vi "KI6221.vi"() -> ()   [LabVIEW 2019] (continued)
      w132 = u16 5 ("Measure Connect LAST")
      w116 = FALSE ("Visible")
      w129 = 0 ("Numeric 2")
      # "SHOW HELP"
      # "Makes 6220 pic NOT visible,\nbecause we don't yet have a\npic... Change with graphics."
      # "Clear setup WIzard"
      n79 = local read "Select the current source model number:"() -> (w119:u16)
      n80 = property on="Verify instruments" class="Bool (strict)"("Visible"=w116) -> ()  [unwired: 2 in, 2 out]
      n81 = property on="BIG DISP OVERLAY" class="Bool (strict)"("Caption.Visible"=w116) -> ()  [unwired: 2 in, 2 out]
      n82 = property on="DUT connect HELP" class="Bool"("Visible"=w116) -> ()  [unwired: 2 in, 2 out]
      n83 = Not(x=w116) -> (.not. x?=w138:bool)
      n84 = property on="DC TABS" class="TabCtl (strict)" props=["Pages", "Value"]() -> (error out=w134:errorcluster, "Pages"=w137:refnum<vi>[])  [unwired: 2 in, 2 out]
      n85 = local read "Power:"() -> (w121:u16)
      n86 = case shown="1" w121 {
        frame 0, Default {
          n87 = local write "INCREMENT"(16.666667) -> ()
        }
        frame 1 {
          n88 = local write "INCREMENT"(20.0) -> ()
        }
      }
      n89 = property on="Voltage\n Compliance" class="DigNum (strict)"("Disabled"=w122) -> ()  [unwired: 2 in, 2 out]
      n90 = property on="SAVE 2" class="Bool"("Disabled"=w129) -> ()  [unwired: 2 in, 2 out]
      n91 = property on="Signal Repetition \nFrequency (Hz)" class="DigNum (strict)"("Disabled"=w122) -> ()  [unwired: 2 in, 2 out]
      n92 = property on="NEW INSTR SETUP" class="Bool"("Disabled"=w129) -> ()  [unwired: 2 in, 2 out]
      n93 = property on="WEB UPDATES" class="Bool (strict)"("Disabled"=w129) -> ()  [unwired: 2 in, 2 out]
      n94 = property on="OPEN" class="Bool (strict)"("Disabled"=w129) -> ()  [unwired: 2 in, 2 out]
      n95 = property on="GENERATE SCPI - ADVANCED" class="Bool"("Disabled"=w129) -> ()  [unwired: 2 in, 2 out]
      n96 = invoke on="Main intro bar" class="Picture" method="Reinit To Default"() -> ()  [unwired: 3 in, 3 out]
      n97 = property on="waveform tabs 2" class="TabCtl (strict)"("Disabled"=w122) -> ()  [unwired: 2 in, 2 out]
      n98 = property on="Waveform Type" class="Ring (strict)"("Disabled"=w122) -> ()  [unwired: 2 in, 2 out]
      n99 = property on="______________________________________________________________________________________________________________" class="Bool (strict)"("Visible"=w138) -> ()  [unwired: 2 in, 2 out]
      n100 = property on="UPLOAD TIME WINDOW" class="Str"("Visible"=w116) -> ()  [unwired: 2 in, 2 out]
      n101 = property class="App"() -> ("Display:Primary Workspace"=w114:T12)  [unwired: 2 in, 2 out]
      n102 = local write "Measure Connect LAST"(w132) -> ()
      n103 = property on="LITTLE DISP OVERLAY" class="Bool (strict)"("Caption.Visible"=w116) -> ()  [unwired: 2 in, 2 out]
      n104 = property on="LOW to EARTH 2" class="Ring (strict)"("Visible"=w116) -> ()  [unwired: 2 in, 2 out]
      n105 = property on="FRONT PANEL 6220" class="Pict"("Visible"=w124) -> ()  [unwired: 2 in, 2 out]
      n106 = property on="ABORT SWEEP" class="Bool (strict)"("Disabled"=u8 2, "Value"=w116) -> ()  [unwired: 2 in, 2 out]
      n107 = property on="STOP 2" class="Bool"("Disabled"=u8 2) -> ()  [unwired: 2 in, 2 out]
      n108 = property on="RUN SWEEP" class="Bool"("Disabled"=u8 0) -> ()  [unwired: 2 in, 2 out]
      n109 = property on="CONTROL" class="Bool (strict)"("Value"=w116) -> ()  [unwired: 2 in, 2 out]
      n110 = property on="DIFF COND DAMPING" class="Bool (strict)"("Visible"=w115, "Value"=w115) -> ()  [unwired: 2 in, 2 out]
      n111 = property on="DAMPING" class="Bool (strict)"("Visible"=w115, "Value"=w115) -> ()  [unwired: 2 in, 2 out]
      n112 = property on="I Sweep V Measure Data" class="Tbl (strict)"("Number of Columns"=u32 4) -> ()  [unwired: 2 in, 2 out]
      n113 = local write "COMM TAB LAST"(w132) -> ()
      n114 = local write "Activate Output"(w124) -> ()
      n115 = Equal?(x=w119, y=u16 1) -> (x = y?=w117:bool)
      n116 = Not(x=w117) -> (.not. x?=w118:bool)
      n117 = property on="connect HELP LINK" class="Bool"("Visible"=w116) -> ()  [unwired: 2 in, 2 out]
      n118 = Unbundle(w114) -> ("Left"=w113:i16, "Top"=w111:i16, "Right"=w112:i16, "Bottom"=w110:i16)
      n119 = property on="Advanced Operation Tab" class="TabCtl (strict)"("Disabled"=w129) -> ()  [unwired: 2 in, 2 out]
      n120 = property on="Src Connect HELP" class="Bool"("Visible"=w116) -> ()  [unwired: 2 in, 2 out]
      n121 = property on="HI IMP devices?" class="Ring (strict)"("Visible"=w116) -> ()  [unwired: 2 in, 2 out]
      n122 = local write "X AXIS LAST -DELTA"(w91) -> ()
      n123 = local write "SETUP YET?"(w129) -> ()
      n124 = property on="BIG DISP Ohm Overlay" class="Bool (strict)"("Caption.Visible"=w116) -> ()  [unwired: 2 in, 2 out]
      n125 = local write "Constant"(0.0 ("Constant")) -> ()
      n126 = property on="RUN 2" class="Bool"("Disabled"=u8 0) -> ()  [unwired: 2 in, 2 out]
      n127 = property on="CAP IN" class="Ring (strict)"("Visible"=w116) -> ()  [unwired: 2 in, 2 out]
      n128 = property on="instrument status" class="Str"("Visible"=w116) -> ()  [unwired: 2 in, 2 out]
      n129 = property on="FRONT PANEL 6220" class="Pict"("Visible"=w117) -> ()  [unwired: 2 in, 2 out]
      n130 = property on="UPLOAD" class="Bool"("Disabled"=w129) -> ()  [unwired: 2 in, 2 out]
      n131 = property on="Main Tabs" class="TabCtl (strict)"("Disabled"=w129) -> ()  [unwired: 2 in, 2 out]
      n132 = local write "X Axis: LAST"(w91) -> ()
      n133 = property on="Knob" class="Knob (strict)"("Visible"=w118) -> ()  [unwired: 2 in, 2 out]
      n134 = property on="RUN" class="Bool"("Disabled"=w129) -> ()  [unwired: 2 in, 2 out]
      n135 = property on="Main intro bar" class="Pict"("Visible"=w116) -> ()  [unwired: 2 in, 2 out]
      n136 = Subtract(x=w111, y=w110) -> (x-y=w108:i16)
      n137 = Subtract(x=w113, y=w112) -> (x-y=w109:i16)
      n138 = property on="EXIT 2" class="Bool (strict)"("Disabled"=w129) -> ()  [unwired: 2 in, 2 out]
      n139 = property on="STOP" class="Bool"("Disabled"=u8 2) -> ()  [unwired: 2 in, 2 out]
      n140 = Absolute Value(x=w108) -> (abs(x)=w92:i16)
      n141 = Absolute Value(x=w109) -> (abs(x)=w93:i16)
      n142 = local write "Scalar?"(w124) -> ()
      n143 = property on="auto test label" class="Str"("Visible"=FALSE) -> ()  [unwired: 2 in, 2 out]
      n144 = property on="Lo earth HELP" class="Bool"("Visible"=w116) -> ()  [unwired: 2 in, 2 out]
      n145 = Subtract(x=w93, y=i16 778 ("Vertical")) -> (x-y=w103:i16)
      n146 = Subtract(x=w92, y=i16 534 ("Vertical")) -> (x-y=w104:i16)
      n147 = Index Array(array=w137, index=1) -> (element=w135:refnum<vi>)
      n148 = property class="Page"(reference=w135, error in=w134, "Page Enabled State"=0 ("index")) -> ()  [unwired: 2 out]
      n149 = Divide(x=w103, y=w105) -> (x/y=w102:dbl)
      n150 = To Word Integer(number=w102) -> (16bit integer=w94:i16)
      n151 = Add(x=w94, y=i16 235 ("Horizontal")) -> (x+y=w97:i16)
      n152 = Divide(x=w104, y=w105) -> (x/y=w101:dbl)
      n153 = To Word Integer(number=w101) -> (16bit integer=w95:i16)
      n154 = Add(x=w95, y=i16 527 ("Vertical")) -> (x+y=w96:i16)
      n155 = Bundle(w97, w96) -> (w98:cluster{i16, i16})  [unwired: 1 in]
      n156 = Control Help Window(0:w98, 1:TRUE ("Show")) -> ()
      "VALID SETUP" <- w116
    }
    frame #4 {
      n157 = while {
        stop <- w192 stop-if-true
        w148 = u32 99 ("y")
        # "set flag for basic operation\nreset."
        # "Previously referenced here.\nUser control hidden in this version."
        # "This is the file save section of the vi. Like file open, it is kind of messy because the cluster has to be populated, but other than that all this section does is save data files and link them to the\nbug report as attachments in case they need sent. Everything else is just sending control values into the correct component of the cluster and writing the cluster to a file as a flattened \nLabVIEW object."
        # "Web updates to the left allows user\nupdates via the ftp server using a \nDOS prompt sys command vi.\n\nBug Report sends comments or bug \ninformation via the SMTP sub vis. \nThis sends email to Keithley when a \nuser has an issue and sends it to us."
        # "The section of the VI below is the file open algorithm. It looks kind of messy, but basically all it does is open the Cluster from the file and load the REFERENCE NODES. For some of the RINGS and other special controls\nsome parsing or calculations has to be done on the cluster data before they can be properly loaded. That is what the subvis are doing."
        # "The modules below execute portions of the while loop code based primarily on case statements from the top row of front panel buttons. SAVE FILE and OPEN FILE are directly below these divided modules."
        # "This code sets sets up the instrument communication controls into VISA resources and then tests to see if \nthey can be correctly located on the bus."
        # "This code call the view SCPI window\nand will save commands to a file."
        # "Update Setup Text String from Verify button."
        # "These are the web help links in the vi. They are all linked into the sub vi"
        # "Above is EXIT vi, loop exit node,\nand 100 msec wait for each loop.\nBelow is the enable/disable for \nenable step source checkbox."
        # "sets demo mode warning to\nvisible when Demo mode is \nactive."
        n158 = case shown="\"Advanced Operation\"" "Main Tabs" {
          frame "General", Default {
            n159 = case shown="\"CONN CONFIG\"" "COMM\nTab Control" {
              selector: "COMM\nTab Control" -> [_ w311 w1093 _]
              frame "STARTUP", Default {
                w235 = u8 0 ("Disabled")
                # "This is the code for the two buttons on the startup panel. LEFT takes you to the connection guide.\nBELOW resets the config variables and then takes you to the config panel.\nRIGHT is NEXT to the config panel"
                n160 = case shown="False" "conn guide" {
                  frame False {
                  }
                  frame True {
                    n161 = local write "CONNECT\nONLY FLAG"(TRUE ("CONNECT\nONLY FLAG")) -> ()
                    n162 = property on="COMM\nTab Control" class="TabCtl (strict)"("Value"=T2."CONN GUIDE" ("COMM\nTab Control")) -> ()  [unwired: 2 in, 2 out]
                  }
                }
                n163 = case shown="False" "NEW INSTR SETUP" {
                  frame False {
                  }
                  frame True {
                    w250 = u16 0 items=["NORMAL OPERATION", "REDUCE C IN 2182A"] ("CAP IN")
                    w254 = i32[] [] ("Disabled Items []")
                    w261 = 0 (".  IP#2")
                    w262 = u16 0 items=["FLOATING OPERATION", "LO TO EARTH CONNECTION"] ("LOW to EARTH 2")
                    w286 = u16 0 items=["SELECT", "6220", "6221"] ("Select the current source model number:")
                    w251 = FALSE ("Visible")
                    n164 = local write "CONNECT\nONLY FLAG"(FALSE ("CONNECT\nONLY FLAG")) -> ()
                    n165 = property on="LOW to EARTH" class="Bool (strict)"("Visible"=w251) -> (error out=w268:errorcluster)  [unwired: 2 in, 1 out]
                    n166 = property on="Select Network Card number:\n(default to zero)" class="DigNum (strict)"(error in=w268, "Visible"=w251) -> (error out=w267:errorcluster)  [unwired: 1 in, 1 out]
                    n167 = local write "NEXT FLAG LAST"(1 ("NEXT FLAG LAST")) -> ()
                    n168 = property on="Select the interface for the 6220/6221:" class="Ring (strict)"("Disabled Items []"=w254) -> ()  [unwired: 2 in, 2 out]
                    n169 = property on="Select the current source model number:" class="Ring (strict)"("Disabled Items []"=w254) -> ()  [unwired: 2 in, 2 out]
                    n170 = local write "NEXT FLAG"(0 ("NEXT FLAG")) -> ()
                    n171 = property on="Select the nanovoltmeter model number:" class="Ring (strict)"("Disabled Items []"=w254) -> ()  [unwired: 2 in, 2 out]
                    n172 = property on="6220 Connect" class="Ring (strict)"("Disabled Items []"=w254) -> ()  [unwired: 2 in, 2 out]
                    n173 = property on="Select GPIB Address number \nof the current source:" class="DigNum (strict)"(error in=w267, "Visible"=w251, "Value"=16 ("Select GPIB Address number \nof the current source:")) -> (error out=w265:errorcluster)  [unwired: 1 in, 1 out]
                    n174 = property on="GPIB 6220 label" class="Str"(error in=w265, "Visible"=w251) -> (error out=w266:errorcluster)  [unwired: 1 in, 1 out]
                    n175 = property on="Select GPIB Board number:\n(default to zero)" class="DigNum (strict)"(error in=w266, "Visible"=w251) -> (error out=w269:errorcluster)  [unwired: 1 in, 1 out]
                    n176 = property on="Select the interface for the 6220/6221:" class="Ring (strict)"(error in=w269, "Visible"=w251) -> (error out=w270:errorcluster)  [unwired: 1 in, 1 out]
                    n177 = property on="sOURCE Connect" class="Ring (strict)"(error in=w270, "Visible"=w251) -> (error out=w271:errorcluster)  [unwired: 1 in, 1 out]
                    n178 = property on="HI IMP devices?" class="Ring (strict)"(error in=w271, "Visible"=w251) -> (error out=w272:errorcluster)  [unwired: 1 in, 1 out]
                    n179 = property on="Main intro bar" class="Pict"(error in=w272, "Visible"=w251) -> (error out=w257:errorcluster)  [unwired: 1 in, 1 out]
                    n180 = property on="Select the current source model number:" class="Ring (strict)"(error in=w257, "Value"=w286) -> (error out=w273:errorcluster)  [unwired: 1 in, 1 out]
                    n181 = property on="Select the nanovoltmeter model number:" class="Ring (strict)"(error in=w273, "Value"=w286) -> (error out=w274:errorcluster)  [unwired: 1 in, 1 out]
                    n182 = property on="Select the interface for the 6220/6221:" class="Ring (strict)"(error in=w274, "Value"=w286) -> (error out=w275:errorcluster)  [unwired: 1 in, 1 out]
                    n183 = property on="HI IMP devices?" class="Ring (strict)"(error in=w275, "Value"=w286) -> (error out=w276:errorcluster)  [unwired: 1 in, 1 out]
                    n184 = property on="6220 Connect" class="Ring (strict)"(error in=w276, "Value"=w286) -> (error out=w277:errorcluster)  [unwired: 1 in, 1 out]
                    n185 = property on="Input instrument IP Address:" class="DigNum (strict)"(error in=w277, "Visible"=w251, "Value"=w261) -> (error out=w278:errorcluster)  [unwired: 1 in, 1 out]
                    n186 = property on=".  IP#4" class="DigNum (strict)"(error in=w278, "Visible"=w251, "Value"=w261) -> (error out=w279:errorcluster)  [unwired: 1 in, 1 out]
                    n187 = property on=".  IP#3" class="DigNum (strict)"(error in=w279, "Visible"=w251, "Value"=w261) -> (error out=w280:errorcluster)  [unwired: 1 in, 1 out]
                    n188 = property on=".  IP#2" class="DigNum (strict)"(error in=w280, "Visible"=w251, "Value"=w261) -> (error out=w264:errorcluster)  [unwired: 1 in, 1 out]
                    n189 = local write "WIZ string"("Instrument Communication Setup Wizard" ("WIZ string")) -> ()
                    n190 = property on="instrument status" class="Str"(error in=w264, "Visible"=w251) -> (error out=w281:errorcluster)  [unwired: 1 in, 1 out]
                    n191 = property on="Verify instruments" class="Bool (strict)"(error in=w281, "Visible"=w251) -> (error out=w263:errorcluster)  [unwired: 1 in, 1 out]
                    n192 = property on="Lo earth HELP" class="Bool"(error in=w263, "Visible"=w251) -> (error out=w282:errorcluster)  [unwired: 1 in, 1 out]
                    n193 = property on="NEXT" class="Bool"("Visible"=TRUE) -> ()  [unwired: 2 in, 2 out]
                    n194 = property on="LOW to EARTH 2" class="Ring (strict)"(error in=w282, "Visible"=w251, "Value"=w262) -> (error out=w283:errorcluster)  [unwired: 1 in, 1 out]
                    n195 = property on="DUT connect HELP" class="Bool"(error in=w283, "Visible"=w251) -> (error out=w284:errorcluster)  [unwired: 1 in, 1 out]
                    n196 = property on="Src Connect HELP" class="Bool"(error in=w284, "Visible"=w251) -> (error out=w285:errorcluster)  [unwired: 1 in, 1 out]
                    n197 = property on="COMM\nTab Control" class="TabCtl (strict)"(error in=w285, "Value"=T2."CONN CONFIG" ("COMM\nTab Control")) -> ()  [unwired: 1 in, 2 out]
                    n198 = local write "SETUP FLAG"(0 ("SETUP FLAG")) -> ()
                    n199 = property on="CAP IN" class="Ring (strict)"("Visible"=w251, "Value"=w250) -> ()  [unwired: 2 in, 2 out]
                  }
                }
                n200 = case shown="True" "EDIT present setup" {
                  frame False {
                  }
                  frame True {
                    w243 = i32[] [0] ("Disabled Items []")
                    w240 = u8 0 ("Disabled")
                    w239 = TRUE ("OK")
                    w244 = TRUE ("Visible")
                    n201 = property on="6220 Connect" class="Ring (strict)"("Visible"=w239, "Disabled"=w240, "Disabled Items []"=w243) -> ()  [unwired: 2 in, 2 out]
                    n202 = property on="HI IMP devices?" class="Ring (strict)"("Visible"=w239, "Disabled"=w240) -> ()  [unwired: 2 in, 2 out]
                    n203 = property on="Power:" class="Ring (strict)"("Visible"=w239, "Disabled"=w240) -> ()  [unwired: 2 in, 2 out]
                    n204 = property on="COMM\nTab Control" class="TabCtl (strict)"("Value"=T2."CONN CONFIG" ("COMM\nTab Control")) -> ()  [unwired: 2 in, 2 out]
                    n205 = property on="Select the nanovoltmeter model number:" class="Ring (strict)"("Visible"=w239, "Disabled"=w240, "Disabled Items []"=w243) -> ()  [unwired: 2 in, 2 out]
                    n206 = local write "SETUP FLAG"(1 ("SETUP FLAG")) -> ()
                    n207 = property on="LOW to EARTH 2" class="Ring (strict)"("Visible"=w239, "Disabled"=w240) -> ()  [unwired: 2 in, 2 out]
                    n208 = property on="Select the current source model number:" class="Ring (strict)"("Visible"=w239, "Disabled"=w240, "Disabled Items []"=w243) -> ()  [unwired: 2 in, 2 out]
                    n209 = property on="CAP IN" class="Ring (strict)"("Visible"=w239, "Disabled"=w240) -> ()  [unwired: 2 in, 2 out]
                    n210 = property on="Select the interface for the 6220/6221:" class="Ring (strict)"("Disabled Items []"=w243, "Disabled"=w240) -> ()  [unwired: 2 in, 2 out]
                    n211 = property on="Verify instruments" class="Bool (strict)"("Visible"=w244) -> ()  [unwired: 2 in, 2 out]
                    n212 = property on="instrument status" class="Str"("Visible"=w244) -> ()  [unwired: 2 in, 2 out]
                    n213 = property on="OK" class="Bool (strict)"("Visible"=w239) -> ()  [unwired: 2 in, 2 out]
                    n214 = property on="CANCEL" class="Bool"("Visible"=w239) -> ()  [unwired: 2 in, 2 out]
                    n215 = property on="NEXT" class="Bool"("Visible"=FALSE) -> ()  [unwired: 2 in, 2 out]
                    n216 = local write "CONNECT\nONLY FLAG"(FALSE ("CONNECT\nONLY FLAG")) -> ()
                    n217 = property on="Main intro bar" class="Pict"("Visible"=w239) -> ()  [unwired: 2 in, 2 out]
                    n218 = property on="Src Connect HELP" class="Bool"("Visible"=w239) -> ()  [unwired: 2 in, 2 out]
                    n219 = property on="Lo earth HELP" class="Bool"("Visible"=w239) -> ()  [unwired: 2 in, 2 out]
                    n220 = property on="DUT connect HELP" class="Bool"("Visible"=w239) -> ()  [unwired: 2 in, 2 out]
                    "WIZ string" <- "Instrument Communication Setup" ("WIZ string")
                  }
                }
                n221 = property on="Main Tabs" class="TabCtl (strict)"("Page Selector Visible"=TRUE) -> ()  [unwired: 2 in, 2 out]
                n222 = property on="EXIT 2" class="Bool (strict)"("Disabled"=w235) -> ()  [unwired: 2 in, 2 out]
                n223 = property on="SAVE 2" class="Bool"("Disabled"=w235) -> ()  [unwired: 2 in, 2 out]
              }
              frame "CONN CONFIG" {
                w303 = FALSE ("Enable")
                w308 = u8 2 ("Disabled")
                # "Graphics Update flag"
                # "This is the code that selects \nthe connection diagrams"
                # "Controls not directly used but in this window."
                # "Calls the help windows for the\nHow do I decide prompts?"
                # "Links the RING Control to the \ncheckbox that we are using."
                # "Returns the settings to their previous value and sends user to the Startup Screen screen."
                # "Sets the Pulse Interval options to select based on power\nfrequency."
                # "Once Connect is selected \nthese other controls and \nlinks become visible."
                # "Sets the config controls with the default values"
                # "Sets the correct interface variables to visible"
                # "Removes tabs so config must\nbe completed before a test \ncan be run."
                # "This code updates the controls and saves the new values as the current settings and the default settings in that box is checked. This executes when OK is clicked."
                n224 = local write "COMM TAB LAST"(w311) -> ()
                n225 = case shown="True" "OK" {
                  frame False {
                  }
                  frame True {
                    n226 = flat-sequence {
                      tunnel: [w999] -> w984
                      tunnel: [w998] -> w983
                      tunnel: [w997] -> w982
                      tunnel: w984 -> [w1054]
                      tunnel: w983 -> [w1049]
                      tunnel: w982 -> [w1044]
                      frame #0 {
                        n227 = property on=".  IP#2" class="DigNum (strict)"() -> ("Value"=w1024:i32)  [unwired: 2 in, 2 out]
                        n228 = property on=".  IP#4" class="DigNum (strict)"() -> ("Value"=w1022:i32)  [unwired: 2 in, 2 out]
                        n229 = property on=".  IP#3" class="DigNum (strict)"() -> ("Value"=w1023:i32)  [unwired: 2 in, 2 out]
                        n230 = property on="at GPIB Address:" class="DigNum (strict)"("Value"="Select GPIB Address number \nof the current source:") -> ()  [unwired: 2 in, 2 out]
                        n231 = property on=".  IP#2" class="DigNum (strict)"("Value"=w1024) -> ()  [unwired: 2 in, 2 out]
                        n232 = property on=".  IP#3 2" class="DigNum (strict)"("Value"=w1023) -> ()  [unwired: 2 in, 2 out]
                        n233 = property on=".  IP#4" class="DigNum (strict)"("Value"=w1022) -> ()  [unwired: 2 in, 2 out]
                        n234 = property on="Select the nanovoltmeter model number:" class="Ring (strict)"() -> ("Value"=w1000:u16)  [unwired: 2 in, 2 out]
                        n235 = property on="Select the current source model number:" class="Ring (strict)"() -> ("Value"=w988:u16)  [unwired: 2 in, 2 out]
                        n236 = Equal?(x=1, y=w988) -> (x = y?=w1014:bool)
                        n237 = property on="Select the interface for the 6220/6221:" class="Ring (strict)"() -> ("Value"=w1008:u16)  [unwired: 2 in, 2 out]
                        n238 = Equal?(x=2, y=w1008) -> (x = y?=w1013:bool)
                        n239 = Or(x=w1014, y=w1013) -> (x .or. y?=w1012:bool)
                        n240 = property on="Default Cluster" class="Clust (strict)"() -> ("Value"=w1017:T8)  [unwired: 2 in, 2 out]
                        n241 = case shown="False" w1012 {
                          tunnel: [0 1] -> w1009
                          frame False {
                          }
                          frame True {
                            # "GPIB"
                          }
                        }
                        n242 = property on="Select Network Card number:\n(default to zero)" class="DigNum (strict)"() -> ("Value"=w1018:i32)  [unwired: 2 in, 2 out]
                        n243 = property on="Select GPIB Address number \nof the current source:" class="DigNum (strict)"() -> ("Value"=w1019:i32)  [unwired: 2 in, 2 out]
                        n244 = property on="Select GPIB Board number:\n(default to zero)" class="DigNum (strict)"() -> ("Value"=w1020:i32)  [unwired: 2 in, 2 out]
                        n245 = property on="DEFAULT setup" class="Bool (strict)"() -> ("Value"=w1026:bool)  [unwired: 2 in, 2 out]
                        n246 = property on="HI IMP devices?" class="Ring (strict)"() -> ("Value"=w1004:u16)  [unwired: 2 in, 2 out]
                        n247 = property on="Source Connect" class="Ring (strict)"() -> ("Value"=w998:u16)  [unwired: 2 in, 2 out]
                        n248 = case shown="2" w988 {
                          tunnel: [2 2 0] -> w1007
                          frame 0, Default {
                          }
                          frame 1 {
                          }
                          frame 2 {
                          }
                        }
                        n249 = property on="LOW to EARTH" class="Bool (strict)"() -> ("Value"=w997:bool)  [unwired: 2 in, 2 out]
                        n250 = property on="Power:" class="Ring (strict)"() -> ("Value"=w1021:u16)  [unwired: 2 in, 2 out]
                        n251 = property on="Input instrument IP Address:" class="DigNum (strict)"() -> ("Value"=w1025:i32)  [unwired: 2 in, 2 out]
                        n252 = property on="Model 6220 or 6221 is connected by:" class="Ring (strict)"("Value"=w1009, "Disabled"=w1007) -> ()  [unwired: 2 in, 2 out]
                        n253 = property on="at instrument IP Address:" class="DigNum (strict)"("Value"=w1025) -> ()  [unwired: 2 in, 2 out]
                        n254 = local write "OK"(FALSE ("OK")) -> ()
                        n255 = Equal?(x=w998, y=u16 2) -> (x = y?=w1006:bool)
                        n256 = Equal?(x=w1004, y=u16 0) -> (x = y?=w1005:bool)
                        n257 = local read "LOW to EARTH 2"() -> (w990:u16)
                        n258 = local read "CAP IN"() -> (w989:u16)
                        n259 = Bundle(cluster=w1017, "Numeric"=w988, "Numeric 2"=w1000, "Numeric 3"=w1008, "Numeric 4"="Input instrument IP Address:", "Numeric 5"=".  IP#2", "Numeric 6"=".  IP#3", "Numeric 7"=".  IP#4", "Numeric 8"=w1018, "Numeric 9"=w1019, "Numeric 10"=w1020, "Numeric 11"=w998, "Numeric 12"=w1004, "Numeric 13"=w1021, "Boolean"=w997, "Numeric 14"=w990, "Numeric 15"=w989) -> (w1016:T8)
                        n260 = case shown="True" w1026 {
                          tunnel: w1016 -> [w1032 w1036]
                          tunnel: [w1032 w1036] -> w1015
                          frame False {
                          }
                          frame True {
                            n261 = property on="Default path" class="Path"() -> ("Value"=w1034:path)  [unwired: 2 in, 2 out]
                            n262 = property on="Default Cluster" class="Clust (strict)"("Value"=w1036) -> ()  [unwired: 2 in, 2 out]
                            n263 = Flatten To String(anything=w1036) -> (data string=w1038:string)  [unwired: 3 in, 2 out]
                            n264 = Build Path(base path=w1034, name or relative path="defaulttest.cfg" ("file path (dialog if empty)")) -> (appended path=w1033:path)
                            n265 = Delete(path (use dialog)=w1033) -> (deleted path=w1039:path, error out=→"error out 2":errorcluster)  [unwired: 4 in, 1 out]
                            n266 = call "WriteToFile.vi"("character string"=w1038, "file path (dialog if empty)"=w1039) -> ()  [unwired: 3 in, 1 out]
                          }
                        }
                        n267 = Equal?(x=w1000, y=u16 3) -> (x = y?=w999:bool)
                        n268 = Equal?(x=w988, y=u16 1) -> (x = y?=w986:bool)
                        n269 = Compound Arithmetic op=AND(w1006, w1005, w999) -> ()  [unwired: 1 out]
                        n270 = property on="Last setup Cluster" class="Clust (strict)"("Value"=w1015) -> ()  [unwired: 2 in, 2 out]
                        n271 = property on="FRONT PANEL 6220" class="Pict"("Visible"=w986) -> ()  [unwired: 2 in, 2 out]
                        n272 = Not(x=w986) -> (.not. x?=w985:bool)
                        n273 = property on="Knob" class="Knob (strict)"("Visible"=w985) -> ()  [unwired: 2 in, 2 out]
                      }
                      frame #1 {
                        # "***CHANGE THIS CONSTANT TO\nTRUE TO ENABLE LO-EARTH\nINTERNAL SHORT"
                        n274 = local read "SETUP FLAG"() -> (w1041:i32)
                        n275 = local write "VALID SETUP"(FALSE ("VALID SETUP")) -> ()
                        n276 = case shown="1" w1041 {
                          tunnel: [T2."CONN GUIDE" ("COMM\nTab Control") T2."STARTUP" ("COMM\nTab Control")] -> w1058
                          frame 0, Default {
                          }
                          frame 1 {
                          }
                        }
                        n277 = local write "SETUP YET?"(0 ("Numeric 2")) -> ()
                        n278 = local read "CAP IN"() -> (w1040:u16)
                        n279 = property on="COMM\nTab Control" class="TabCtl (strict)"("Value"=w1058) -> ()  [unwired: 2 in, 2 out]
                        n280 = case shown="True" w1054 {
                          tunnel: [w1070 ":SYST:COMM:SERIal:SEND \"SYST:FFIL " ("string")] -> w1055
                          tunnel: w1040 -> [_ w1074]
                          tunnel: [w1070 w1073] -> w1053
                          tunnel: [w1070 "\"" ("string")] -> w1052
                          tunnel: [w1070 "\n"] -> w1051
                          frame False {
                            w1070 = ""
                          }
                          frame True {
                            n281 = case shown="1" w1074 {
                              tunnel: ["ON" ("string") "OFF" ("string")] -> w1073
                              frame 0, Default {
                              }
                              frame 1 {
                              }
                            }
                          }
                        }
                        n282 = case shown="2, Default" w1049 {
                          tunnel: ["GUAR" ("string") "OLOW" ("string")] -> w1048
                          frame 2, Default {
                          }
                          frame 1 {
                          }
                        }
                        n283 = case shown="True" "Case Constant\n(See Context Help)" {
                          tunnel: [w1061 w1065] -> w1047
                          tunnel: [w1061 ":outp:lte " ("string")] -> w1046
                          tunnel: w1044 -> [_ w1063]
                          tunnel: [w1061 "\n"] -> w1042
                          frame False {
                            w1061 = ""
                          }
                          frame True {
                            n284 = case shown="True" w1063 {
                              tunnel: ["OFF" ("string") "ON" ("string")] -> w1065
                              frame False {
                              }
                              frame True {
                              }
                            }
                          }
                        }
                        n285 = Concatenate Strings(w1055, w1053, w1052, w1051, ":OUTP:ISH " ("string"), w1048, w1042, w1046, w1047) -> (→"Setup String":string)
                      }
                    }
                  }
                }
                n286 = case shown="True" "default use 2" {
                  frame False {
                  }
                  frame True {
                    n287 = flat-sequence {
                      frame #0 {
                        n288 = property on="Default Cluster" class="Clust (strict)"() -> ("Value"=w932:T8)  [unwired: 2 in, 2 out]
                        n289 = Unbundle(w932) -> ("Numeric"=w923:i32, "Numeric 2"=w931:i32, "Numeric 3"=w938:i32, "Numeric 4"=w940:i32, "Numeric 5"=w941:i32, "Numeric 6"=w942:i32, "Numeric 7"=w943:i32, "Numeric 8"=w930:i32, "Numeric 9"=w944:i32, "Numeric 10"=w929:i32, "Numeric 11"=w928:i32, "Numeric 12"=w927:i32, "Numeric 13"=w926:i32, "Boolean"=w925:bool, "Numeric 14"=w922:u16, "Numeric 15"=w921:u16)
                        n290 = property on="at instrument IP Address:" class="DigNum (strict)"("Value"=w940) -> ()  [unwired: 2 in, 2 out]
                        n291 = property on=".  IP#3 2" class="DigNum (strict)"("Value"=w942) -> ()  [unwired: 2 in, 2 out]
                        n292 = Equal?(x=1, y=w923) -> (x = y?=w937:bool)
                        n293 = Equal?(x=2, y=w938) -> (x = y?=w936:bool)
                        n294 = Or(x=w937, y=w936) -> (x .or. y?=w935:bool)
                        n295 = property on=".  IP#2" class="DigNum (strict)"("Value"=w941) -> ()  [unwired: 2 in, 2 out]
                        n296 = property on=".  IP#4" class="DigNum (strict)"("Value"=w943) -> ()  [unwired: 2 in, 2 out]
                        n297 = case shown="True" w935 {
                          tunnel: [0 1] -> w939
                          frame False {
                          }
                          frame True {
                            # "GPIB"
                          }
                        }
                        n298 = property on="at GPIB Address:" class="DigNum (strict)"("Value"=w944) -> ()  [unwired: 2 in, 2 out]
                        n299 = case shown="2" w923 {
                          tunnel: [2 2 0] -> w924
                          frame 0, Default {
                          }
                          frame 1 {
                          }
                          frame 2 {
                          }
                        }
                        n300 = property on="Model 6220 or 6221 is connected by:" class="Ring (strict)"("Value"=w939, "Disabled"=w924) -> ()  [unwired: 2 in, 2 out]
                        n301 = property on="Select the current source model number:" class="Ring (strict)"("Value"=w923) -> ()  [unwired: 2 in, 2 out]
                        n302 = property on="Select the nanovoltmeter model number:" class="Ring (strict)"("Value"=w931) -> ()  [unwired: 2 in, 2 out]
                        n303 = property on="Select the interface for the 6220/6221:" class="Ring (strict)"("Value"=w938) -> ()  [unwired: 2 in, 2 out]
                        n304 = property on="Input instrument IP Address:" class="DigNum (strict)"("Value"=w940) -> ()  [unwired: 2 in, 2 out]
                        n305 = property on=".  IP#2" class="DigNum (strict)"("Value"=w941) -> ()  [unwired: 2 in, 2 out]
                        n306 = property on=".  IP#3" class="DigNum (strict)"("Value"=w942) -> ()  [unwired: 2 in, 2 out]
                        n307 = property on=".  IP#4" class="DigNum (strict)"("Value"=w943) -> ()  [unwired: 2 in, 2 out]
                        n308 = property on="Select GPIB Address number \nof the current source:" class="DigNum (strict)"("Value"=w944) -> ()  [unwired: 2 in, 2 out]
                        n309 = property on="Select GPIB Board number:\n(default to zero)" class="DigNum (strict)"("Value"=w929) -> ()  [unwired: 2 in, 2 out]
                        n310 = property on="Select Network Card number:\n(default to zero)" class="DigNum (strict)"("Value"=w930) -> ()  [unwired: 2 in, 2 out]
                        n311 = local write "LOW to EARTH 2"(w922) -> ()
                        n312 = local write "CAP IN"(w921) -> ()
                        n313 = property on="LOW to EARTH" class="Bool (strict)"("Value"=w925) -> ()  [unwired: 2 in, 2 out]
                        n314 = property on="The current source is set up for easy cabling in STANDARD CONNECTIONS mode. This \nallows for many versatile measurement setups. However, with high impedance\ndevices or with significant cable capacitance the RC product in the circuit can impact the \ninstrument's risetime for some tests. If you would like to make GUARDED CONNECTIONS\nbecause of the RC present in your test system or for any other reason select GUARDED\nCONNECTIONS below, otherwise use STANDARD CONNECTIONS." class="Ring (strict)"("Value"=w928) -> ()  [unwired: 2 in, 2 out]
                        n315 = property on="HI IMP devices?" class="Ring (strict)"("Value"=w927) -> ()  [unwired: 2 in, 2 out]
                        n316 = property on="Power:" class="Ring (strict)"("Value"=w926) -> ()  [unwired: 2 in, 2 out]
                      }
                      frame #1 {
                        n317 = local write "VALID SETUP"(FALSE ("VALID SETUP")) -> ()
                        n318 = local write "SETUP YET?"(0 ("Numeric 2")) -> ()
                      }
                    }
                  }
                }
                n319 = case shown="True" "Case Constant\n(See Context Help) 2" {
                  frame False {
                  }
                  frame True {
                    w917 = TRUE
                    n320 = property on="HI IMP devices?" class="Ring (strict)"("Visible"=w917) -> ()  [unwired: 2 in, 2 out]
                    n321 = property on="LOW to EARTH 2" class="Ring (strict)"("Visible"=w917) -> ()  [unwired: 2 in, 2 out]
                    n322 = property on="CAP IN" class="Ring (strict)"("Visible"=w917) -> ()  [unwired: 2 in, 2 out]
                    n323 = property on="OK" class="Bool (strict)"("Disabled"=u8 0) -> ()  [unwired: 2 in, 2 out]
                  }
                }
                n324 = Not Equal To 0?(x="LOW to EARTH 2") -> (x != 0?=w317:bool)
                n325 = local write "LOW to EARTH"(w317) -> ()
                n326 = case shown="0, Default" "Power:" {
                  frame 0, Default {
                    n327 = local write "INCREMENT"(16.666667) -> ()
                  }
                  frame 1 {
                    "INCREMENT" <- 20.0
                  }
                }
                n328 = Not Equal?(x="6220 Connect LAST", y="6220 Connect") -> (x != y?=w309:bool)
                n329 = local read "Select the nanovoltmeter model number:"() -> (w289:u16)
                n330 = Not Equal?(x="LOW2EARTH LAST", y="LOW to EARTH 2") -> (x != y?=w316:bool)
                n331 = Not Equal?(x="Measure Connect LAST", y="HI IMP devices?") -> (x != y?=w315:bool)
                n332 = Not Equal?(x="nv METER LAST", y=w289) -> (x != y?=w288:bool)
                n333 = Compound Arithmetic op=OR(w316, w315, w309, w288) -> (w312:bool)
                n334 = property on="Main Tabs" class="TabCtl (strict)"("Page Selector Visible"=FALSE) -> ()  [unwired: 2 in, 2 out]
                n335 = Decrement(x="6220 Connect") -> (x-1=w293:u16)
                n336 = case shown="True" w312 {
                  tunnel: "LOW to EARTH 2" -> [_ w891]
                  tunnel: "HI IMP devices?" -> [_ w890]
                  tunnel: "6220 Connect" -> [_ w892]
                  tunnel: w289 -> [_ w888]
                  frame False {
                  }
                  frame True {
                    n337 = local read "Default path"() -> (w900:path)
                    n338 = Equal To 0?(x=w892) -> (x = 0?=w896:bool)
                    n339 = case shown="False" w896 {
                      tunnel: [w909 "0" ("string")] -> w895
                      tunnel: [w907 "0" ("string")] -> w894
                      tunnel: [w905 "0" ("string")] -> w893
                      tunnel: w892 -> [w910 _]
                      tunnel: w891 -> [w908 _]
                      tunnel: w890 -> [w906 _]
                      tunnel: w888 -> [w904 _]
                      frame False {
                        n340 = Number To Decimal String(number=w908) -> (decimal integer string=w907:string)  [unwired: 1 in]
                        n341 = case shown="1" w904 {
                          tunnel: w906 -> [_ w913]
                          tunnel: ["2" w912] -> w905
                          frame 1 {
                          }
                          frame 2, Default {
                            n342 = Number To Decimal String(number=w913) -> (decimal integer string=w912:string)  [unwired: 1 in]
                          }
                        }
                        n343 = Number To Decimal String(number=w910) -> (decimal integer string=w909:string)  [unwired: 1 in]
                      }
                      frame True {
                      }
                    }
                    n344 = local write "Measure Connect LAST"(w890) -> ()
                    n345 = local write "LOW2EARTH LAST"(w891) -> ()
                    n346 = local write "6220 Connect LAST"(w892) -> ()
                    n347 = Concatenate Strings("Connect" ("string"), w895, w894, w893, ".png" ("string")) -> (w899:string)
                    n348 = Build Path(base path=w900, name or relative path=w899) -> (appended path=w901:path)
                    n349 = call <vilib>:"Read PNG File.vi"("path to PNG file"=w901) -> ("error out"=→"error out 3":errorcluster, "image data"=w902:T13)  [unwired: 8 in, 1 out]
                    n350 = call <vilib>:"Draw Flattened Pixmap.vi"("image data"=w902) -> ("new picture"=w889:picture)  [unwired: 8 in]
                    n351 = local write "Main intro bar"(w889) -> ()
                    n352 = local write "nv METER LAST"(w888) -> ()
                  }
                }
                n353 = case shown="True" "CANCEL" {
                  frame False {
                  }
                  frame True {
                    n354 = flat-sequence {
                      frame #0 {
                        n355 = property on="Last setup Cluster" class="Clust (strict)"() -> ("Value"=w954:T8)  [unwired: 2 in, 2 out]
                        n356 = Unbundle(w954) -> ("Numeric"=w974:i32, "Numeric 2"=w955:i32, "Numeric 3"=w970:i32, "Numeric 4"=w962:i32, "Numeric 5"=w963:i32, "Numeric 6"=w964:i32, "Numeric 7"=w965:i32, "Numeric 8"=w956:i32, "Numeric 9"=w966:i32, "Numeric 10"=w957:i32, "Numeric 11"=w958:i32, "Numeric 12"=w959:i32, "Numeric 13"=w960:i32, "Boolean"=w961:bool, "Numeric 14"=w953:u16, "Numeric 15"=w952:u16)
                        n357 = local write "CAP IN"(w952) -> ()
                        n358 = Equal?(x=1, y=w974) -> (x = y?=w967:bool)
                        n359 = Equal?(x=2, y=w970) -> (x = y?=w973:bool)
                        n360 = Or(x=w967, y=w973) -> (x .or. y?=w971:bool)
                        n361 = property on="at instrument IP Address:" class="DigNum (strict)"("Value"=w962) -> ()  [unwired: 2 in, 2 out]
                        n362 = property on=".  IP#2" class="DigNum (strict)"("Value"=w963) -> ()  [unwired: 2 in, 2 out]
                        n363 = property on=".  IP#3 2" class="DigNum (strict)"("Value"=w964) -> ()  [unwired: 2 in, 2 out]
                        n364 = property on=".  IP#4" class="DigNum (strict)"("Value"=w965) -> ()  [unwired: 2 in, 2 out]
                        n365 = property on="at GPIB Address:" class="DigNum (strict)"("Value"=w966) -> ()  [unwired: 2 in, 2 out]
                        n366 = case shown="True" w971 {
                          tunnel: [0 1] -> w972
                          frame False {
                          }
                          frame True {
                            # "GPIB"
                          }
                        }
                        n367 = local write "LOW to EARTH 2"(w953) -> ()
                        n368 = property on="Select the current source model number:" class="Ring (strict)"("Value"=w974) -> ()  [unwired: 2 in, 2 out]
                        n369 = property on="Select the nanovoltmeter model number:" class="Ring (strict)"("Value"=w955) -> ()  [unwired: 2 in, 2 out]
                        n370 = property on="Select the interface for the 6220/6221:" class="Ring (strict)"("Value"=w970) -> ()  [unwired: 2 in, 2 out]
                        n371 = property on="Input instrument IP Address:" class="DigNum (strict)"("Value"=w962) -> ()  [unwired: 2 in, 2 out]
                        n372 = property on=".  IP#2" class="DigNum (strict)"("Value"=w963) -> ()  [unwired: 2 in, 2 out]
                        n373 = property on="Select Network Card number:\n(default to zero)" class="DigNum (strict)"("Value"=w956) -> ()  [unwired: 2 in, 2 out]
                        n374 = property on="Select GPIB Address number \nof the current source:" class="DigNum (strict)"("Value"=w966) -> ()  [unwired: 2 in, 2 out]
                        n375 = case shown="2" w974 {
                          tunnel: [2 2 0] -> w975
                          frame 0, Default {
                          }
                          frame 1 {
                          }
                          frame 2 {
                          }
                        }
                        n376 = property on=".  IP#3" class="DigNum (strict)"("Value"=w964) -> ()  [unwired: 2 in, 2 out]
                        n377 = property on="Model 6220 or 6221 is connected by:" class="Ring (strict)"("Value"=w972, "Disabled"=w975) -> ()  [unwired: 2 in, 2 out]
                        n378 = property on="Select GPIB Board number:\n(default to zero)" class="DigNum (strict)"("Value"=w957) -> ()  [unwired: 2 in, 2 out]
                        n379 = property on=".  IP#4" class="DigNum (strict)"("Value"=w965) -> ()  [unwired: 2 in, 2 out]
                        n380 = property on="The current source is set up for easy cabling in STANDARD CONNECTIONS mode. This \nallows for many versatile measurement setups. However, with high impedance\ndevices or with significant cable capacitance the RC product in the circuit can impact the \ninstrument's risetime for some tests. If you would like to make GUARDED CONNECTIONS\nbecause of the RC present in your test system or for any other reason select GUARDED\nCONNECTIONS below, otherwise use STANDARD CONNECTIONS." class="Ring (strict)"("Value"=w958) -> ()  [unwired: 2 in, 2 out]
                        n381 = property on="HI IMP devices?" class="Ring (strict)"("Value"=w959) -> ()  [unwired: 2 in, 2 out]
                        n382 = property on="LOW to EARTH" class="Bool (strict)"("Value"=w961) -> ()  [unwired: 2 in, 2 out]
                        n383 = property on="Power:" class="Ring (strict)"("Value"=w960) -> ()  [unwired: 2 in, 2 out]
                      }
                      frame #1 {
                        n384 = property on="COMM\nTab Control" class="TabCtl (strict)"("Value"=T2."STARTUP" ("COMM\nTab Control")) -> ()  [unwired: 2 in, 2 out]
                      }
                    }
                  }
                }
                n385 = property on="EXIT 2" class="Bool (strict)"("Disabled"=w308) -> ()  [unwired: 2 in, 2 out]
                n386 = property on="SAVE 2" class="Bool"("Disabled"=w308) -> ()  [unwired: 2 in, 2 out]
                n387 = local read "Select the nanovoltmeter model number:"() -> (w292:u16)
                n388 = local read "Default path"() -> (w298:path)
                n389 = case shown="0, Default" "SETUP FLAG" {
                  tunnel: "NEXT" -> [w393 _]
                  tunnel: "BACK" -> [w392 _]
                  tunnel: w298 -> [w381 _]
                  tunnel: w292 -> [w380 w876]
                  tunnel: w293 -> [w379 _]
                  tunnel: "CAP IN" -> [w378 _]
                  tunnel: "HI IMP devices?" -> [w377 _]
                  tunnel: "LOW to EARTH 2" -> [w376 _]
                  frame 0, Default {
                    # "WIZARD"
                    n390 = local read "Select the interface for the 6220/6221:"() -> (w389:u16)
                    n391 = local read "Select the current source model number:"() -> (w388:u16)
                    n392 = local read "Select the nanovoltmeter model number:"() -> (w387:u16)
                    n393 = local read "6220 Connect"() -> (w386:u16)
                    n394 = case shown="True" w393 {
                      tunnel: "NEXT FLAG" -> [_ w866]
                      frame False {
                      }
                      frame True {
                        n395 = Increment(x=w866) -> (x+1=w865:i32)
                        n396 = local write "NEXT FLAG"(w865) -> ()
                        n397 = local read "DEMO MODE"() -> (w860:bool)
                        n398 = Not(x=w860) -> (.not. x?=w857:bool)
                        n399 = Equal?(x=w866, y=4) -> (x = y?=w861:bool)
                        n400 = Equal?(x=w865, y=5) -> (x = y?=w862:bool)
                        n401 = And(x=w861, y=w862) -> (x .and. y?=w859:bool)
                        n402 = And(x=w857, y=w859) -> (x .and. y?=w858:bool)
                        n403 = case shown="True" w858 {
                          frame False {
                          }
                          frame True {
                            w867 = u8 2 ("Disabled")
                            n404 = local write "Verify instruments"(TRUE ("Verify instruments")) -> ()
                            n405 = property on="NEXT" class="Bool"("Disabled"=w867) -> ()  [unwired: 2 in, 2 out]
                            n406 = property on="BACK" class="Bool"("Disabled"=w867) -> ()  [unwired: 2 in, 2 out]
                          }
                        }
                      }
                    }
                    n407 = case shown="True" w392 {
                      tunnel: "NEXT FLAG" -> [_ w856]
                      frame False {
                      }
                      frame True {
                        n408 = Decrement(x=w856) -> (x-1=w855:i32)
                        n409 = local write "NEXT FLAG"(w855) -> ()
                      }
                    }
                    n410 = Not Equal?(x="NEXT FLAG LAST", y="NEXT FLAG") -> (x != y?=w390:bool)
                    n411 = Compound Arithmetic op=ADD(w389, w388, w387, w386) -> (w382:u16)
                    n412 = Not Equal?(x="SUM LAST", y=w382) -> (x != y?=w384:bool)
                    n413 = Or(x=w384, y=w390) -> (x .or. y?=w385:bool)
                    n414 = case shown="True" w385 {
                      tunnel: "NEXT FLAG" -> [_ w421]
                      tunnel: w382 -> [_ w419]
                      tunnel: "NEXT FLAG LAST" -> [_ w414]
                      tunnel: w381 -> [_ w412]
                      tunnel: w380 -> [_ w401]
                      tunnel: w379 -> [_ w411]
                      tunnel: w378 -> [_ w410]
                      tunnel: w377 -> [_ w409]
                      tunnel: w376 -> [_ w408]
                      tunnel: "NEXT FLAG LAST" -> [_ w399]
                      frame False {
                      }
                      frame True {
                        w405 = FALSE ("Visible")
                        n415 = local write "NEXT FLAG LAST"(w421) -> ()
                        n416 = local write "SUM LAST"(w419) -> ()
                        n417 = local read "Select the interface for the 6220/6221:"() -> (w424:u16)
                        n418 = local read "Select the current source model number:"() -> (w415:u16)
                        n419 = case shown="9" w421 {
                          selector: w421 -> [_ _ w543 _ _ _ _ _ _ _]
                          tunnel: [FALSE ("VALID SETUP") TRUE ("VALID SETUP") TRUE ("VALID SETUP") TRUE ("VALID SETUP") TRUE ("VALID SETUP") TRUE ("VALID SETUP") TRUE ("VALID SETUP") TRUE ("VALID SETUP") TRUE ("VALID SETUP") TRUE ("VALID SETUP")] -> w444
                          tunnel: [2 ("Numeric 2") 0 ("Numeric 2") 2 ("Numeric 2") 2 ("Numeric 2") 2 ("Numeric 2") 2 ("Numeric 2") 2 ("Numeric 2") 2 ("Numeric 2") 2 ("Numeric 2") 2 ("Numeric 2")] -> w443
                          tunnel: [FALSE ("VALID SETUP") FALSE ("VALID SETUP") FALSE ("VALID SETUP") FALSE ("VALID SETUP") w641 w678 w717 w752 w790 w828] -> w417
                          tunnel: [2 ("Numeric 2") 0 ("Numeric 2") 0 ("Numeric 2") 0 ("Numeric 2") 2 ("Numeric 2") 2 ("Numeric 2") 2 ("Numeric 2") 2 ("Numeric 2") 2 ("Numeric 2") 2 ("Numeric 2")] -> w440
                          tunnel: [TRUE ("VALID SETUP") TRUE ("VALID SETUP") TRUE ("VALID SETUP") TRUE ("VALID SETUP") TRUE ("VALID SETUP") TRUE ("VALID SETUP") TRUE ("VALID SETUP") TRUE ("VALID SETUP") TRUE ("VALID SETUP") TRUE ("VALID SETUP")] -> w425
                          tunnel: [0 ("Numeric 2") 2 ("Numeric 2") 2 ("Numeric 2") 2 ("Numeric 2") 2 ("Numeric 2") 2 ("Numeric 2") 2 ("Numeric 2") 2 ("Numeric 2") 2 ("Numeric 2") 2 ("Numeric 2")] -> w445
                          tunnel: [w467 FALSE ("VALID SETUP") w575 TRUE ("VALID SETUP") TRUE ("VALID SETUP") TRUE ("VALID SETUP") TRUE ("VALID SETUP") TRUE ("VALID SETUP") TRUE ("VALID SETUP") TRUE ("VALID SETUP")] -> w442
                          tunnel: [2 ("Numeric 2") 0 ("Numeric 2") 0 ("Numeric 2") 2 ("Numeric 2") 2 ("Numeric 2") 2 ("Numeric 2") 2 ("Numeric 2") 2 ("Numeric 2") 2 ("Numeric 2") 2 ("Numeric 2")] -> w441
                          tunnel: [FALSE ("VALID SETUP") FALSE ("VALID SETUP") FALSE ("VALID SETUP") FALSE ("VALID SETUP") w640 w676 w716 w751 w789 w827] -> w439
                          tunnel: [2 ("Numeric 2") 2 ("Numeric 2") 2 ("Numeric 2") 2 ("Numeric 2") 0 ("Numeric 2") 2 ("Numeric 2") 2 ("Numeric 2") 2 ("Numeric 2") 2 ("Numeric 2") 2 ("Numeric 2")] -> w438
                          tunnel: [FALSE ("VALID SETUP") FALSE ("VALID SETUP") FALSE ("VALID SETUP") FALSE ("VALID SETUP") FALSE ("VALID SETUP") TRUE ("VALID SETUP") TRUE ("VALID SETUP") TRUE ("VALID SETUP") TRUE ("VALID SETUP") TRUE ("VALID SETUP")] -> w418
                          tunnel: [2 ("Numeric 2") 2 ("Numeric 2") 2 ("Numeric 2") 2 ("Numeric 2") 2 ("Numeric 2") 0 ("Numeric 2") 2 ("Numeric 2") 2 ("Numeric 2") 2 ("Numeric 2") 2 ("Numeric 2")] -> w437
                          tunnel: [FALSE ("VALID SETUP") w505 FALSE ("VALID SETUP") w605 w641 w678 w717 w752 w790 w828] -> w416
                          tunnel: [2 ("Numeric 2") 0 ("Numeric 2") 0 ("Numeric 2") 2 ("Numeric 2") 0 ("Numeric 2") 2 ("Numeric 2") 2 ("Numeric 2") 2 ("Numeric 2") 2 ("Numeric 2") 2 ("Numeric 2")] -> w436
                          tunnel: [FALSE ("VALID SETUP") FALSE ("VALID SETUP") FALSE ("VALID SETUP") w604 w640 w676 w716 w751 w789 w827] -> w435
                          tunnel: [2 ("Numeric 2") 0 ("Numeric 2") 0 ("Numeric 2") 0 ("Numeric 2") 2 ("Numeric 2") 2 ("Numeric 2") 2 ("Numeric 2") 2 ("Numeric 2") 2 ("Numeric 2") 2 ("Numeric 2")] -> w434
                          tunnel: [FALSE ("VALID SETUP") FALSE ("VALID SETUP") FALSE ("VALID SETUP") w604 w640 w676 w716 w751 w789 w827] -> w433
                          tunnel: [2 ("Numeric 2") 2 ("Numeric 2") 2 ("Numeric 2") 0 ("Numeric 2") 2 ("Numeric 2") 2 ("Numeric 2") 2 ("Numeric 2") 2 ("Numeric 2") 2 ("Numeric 2") 2 ("Numeric 2")] -> w432
                          tunnel: [FALSE ("VALID SETUP") FALSE ("VALID SETUP") FALSE ("VALID SETUP") w604 w640 w676 w716 w751 w789 w827] -> w431
                          tunnel: [2 ("Numeric 2") 2 ("Numeric 2") 2 ("Numeric 2") 0 ("Numeric 2") 2 ("Numeric 2") 2 ("Numeric 2") 2 ("Numeric 2") 2 ("Numeric 2") 2 ("Numeric 2") 2 ("Numeric 2")] -> w430
                          tunnel: [FALSE ("VALID SETUP") FALSE ("VALID SETUP") FALSE ("VALID SETUP") w604 w640 w676 w716 w751 w789 w827] -> w429
                          tunnel: [2 ("Numeric 2") 0 ("Numeric 2") 0 ("Numeric 2") 0 ("Numeric 2") 2 ("Numeric 2") 2 ("Numeric 2") 2 ("Numeric 2") 2 ("Numeric 2") 2 ("Numeric 2") 2 ("Numeric 2")] -> w428
                          tunnel: [FALSE ("VALID SETUP") FALSE ("VALID SETUP") FALSE ("VALID SETUP") FALSE ("VALID SETUP") FALSE ("VALID SETUP") FALSE ("VALID SETUP") FALSE ("VALID SETUP") TRUE ("VALID SETUP") TRUE ("VALID SETUP") TRUE ("VALID SETUP")] -> w403
                          tunnel: [2 ("Numeric 2") 0 ("Numeric 2") 0 ("Numeric 2") 0 ("Numeric 2") 2 ("Numeric 2") 0 ("Numeric 2") 2 ("Numeric 2") 2 ("Numeric 2") 0 ("Numeric 2") 2 ("Numeric 2")] -> w413
                          tunnel: [FALSE ("VALID SETUP") FALSE ("VALID SETUP") FALSE ("VALID SETUP") FALSE ("VALID SETUP") FALSE ("VALID SETUP") FALSE ("VALID SETUP") FALSE ("VALID SETUP") FALSE ("VALID SETUP") TRUE ("VALID SETUP") TRUE ("VALID SETUP")] -> w423
                          tunnel: [2 ("Numeric 2") 2 ("Numeric 2") 2 ("Numeric 2") 2 ("Numeric 2") 2 ("Numeric 2") 2 ("Numeric 2") 2 ("Numeric 2") 0 ("Numeric 2") 2 ("Numeric 2") 2 ("Numeric 2")] -> w427
                          tunnel: [FALSE ("VALID SETUP") w506 FALSE ("VALID SETUP") FALSE ("VALID SETUP") FALSE ("VALID SETUP") FALSE ("VALID SETUP") TRUE ("VALID SETUP") TRUE ("VALID SETUP") TRUE ("VALID SETUP") TRUE ("VALID SETUP")] -> w422
                          tunnel: [2 ("Numeric 2") 0 ("Numeric 2") 0 ("Numeric 2") 0 ("Numeric 2") 2 ("Numeric 2") 2 ("Numeric 2") 0 ("Numeric 2") 2 ("Numeric 2") 2 ("Numeric 2") 2 ("Numeric 2")] -> w426
                          tunnel: w424 -> [_ _ w549 w601 w642 w677 w718 w753 w791 w829]
                          tunnel: [w470 w508 w551 0 0 w675 w711 0 0 0] -> w398
                          tunnel: [TRUE ("VALID SETUP") w506 FALSE ("VALID SETUP") FALSE ("VALID SETUP") FALSE ("VALID SETUP") FALSE ("VALID SETUP") FALSE ("VALID SETUP") FALSE ("VALID SETUP") FALSE ("VALID SETUP") FALSE ("VALID SETUP")] -> w420
                          tunnel: w415 -> [_ _ w548 w598 _ _ _ _ _ _]
                          tunnel: w414 -> [_ _ w542 _ _ _ _ _ _ _]
                          tunnel: [FALSE ("VALID SETUP") FALSE ("VALID SETUP") FALSE ("VALID SETUP") FALSE ("VALID SETUP") FALSE ("VALID SETUP") FALSE ("VALID SETUP") TRUE ("VALID SETUP") w744 w786 FALSE ("VALID SETUP")] -> w407
                          tunnel: [0 ("wizard?") 0 ("wizard?") 0 ("wizard?") 0 ("wizard?") 0 ("wizard?") 0 ("wizard?") 0 ("wizard?") 2 ("wizard?") 3 ("wizard?") 0 ("wizard?")] -> w406
                          tunnel: [2 2 2 2 2 2 2 2 2 0] -> w404
                          tunnel: [FALSE ("VALID SETUP") FALSE ("VALID SETUP") FALSE ("VALID SETUP") FALSE ("VALID SETUP") FALSE ("VALID SETUP") FALSE ("VALID SETUP") FALSE ("VALID SETUP") FALSE ("VALID SETUP") w783 TRUE ("VALID SETUP")] -> w394
                          tunnel: w401 -> [_ _ _ _ _ _ _ _ w782 _]
                          tunnel: w399 -> [_ _ _ _ _ _ _ w745 w781 _]
                          frame 0, Default {
                            w467 = FALSE ("VALID SETUP")
                            n420 = local read "Select the current source model number:"() -> (w474:u16)
                            n421 = Equal To 0?(x=w474) -> (x = 0?=w473:bool)
                            n422 = property on="GPIB 6220 label" class="Str"("Visible"=w467) -> ()  [unwired: 2 in, 2 out]
                            n423 = Select(t=i16 2, s=w473, f=0 ("Numeric 2")) -> (s? t:f=w470:i32)
                          }
                          frame 1 {
                            w505 = FALSE ("VALID SETUP")
                            w506 = FALSE ("VALID SETUP")
                            n424 = local read "Select the nanovoltmeter model number:"() -> (w507:u16)
                            n425 = property on="GPIB 6220 label" class="Str"("Visible"=w505) -> ()  [unwired: 2 in, 2 out]
                            n426 = Equal To 0?(x=w507) -> (x = 0?=w511:bool)
                            n427 = Select(t=i16 2, s=w511, f=0 ("Numeric 2")) -> (s? t:f=w508:i32)
                          }
                          frame 2 {
                            n428 = Equal To 0?(x=w549) -> (x = 0?=w547:bool)
                            n429 = case shown="1" w548 {
                              tunnel: [TRUE ("VALID SETUP") FALSE ("VALID SETUP")] -> w575
                              tunnel: [FALSE ("VALID SETUP") TRUE ("VALID SETUP")] -> w544
                              frame 2, Default {
                              }
                              frame 1 {
                              }
                            }
                            n430 = Not(x=w544) -> (.not. x?=w545:bool)
                            n431 = And(x=w545, y=w547) -> (x .and. y?=w546:bool)
                            n432 = case shown="True" w544 {
                              tunnel: w543 -> [_ w584]
                              tunnel: w542 -> [_ w582]
                              frame False {
                              }
                              frame True {
                                n433 = case shown="1" w582 {
                                tunnel: w584 -> [w585 w588]
                                tunnel: [w586 w587] -> w583
                                frame 3, Default {
                                n434 = Decrement(x=w585) -> (x-1=w586:i32)
                                }
                                frame 1 {
                                n435 = Increment(x=w588) -> (x+1=w587:i32)
                                }
                                }
                                n436 = local write "NEXT FLAG"(w583) -> ()
                              }
                            }
                            n437 = property on="GPIB 6220 label" class="Str"("Visible"=w544) -> ()  [unwired: 2 in, 2 out]
                            n438 = Select(t=i16 2, s=w546, f=0 ("Numeric 2")) -> (s? t:f=w551:i32)
                          }
                          frame 3 {
